vi "ExposeFromObjectMap.vi"(8 "Allow Variant Values (f)":bool, 10 "Object Map":T1[](array[typedef]), 11 "Type (or value to update)":variant) -> (3 "Value":variant)   [LabVIEW 2017]
uses:
  ExposeObjectMapNamepathData.ctl
  ExposeObjectMapDataTypeEnum.ctl
  ExposeObjectMapContainerTypeEnum.ctl
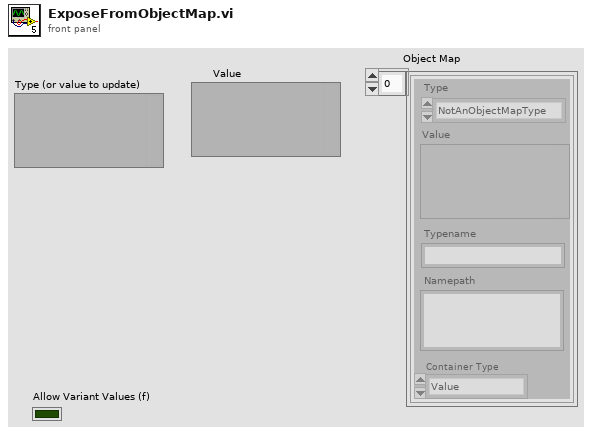
[diagram p1: front panel]
types:
  T1 = typedef "ExposeObjectMapNamepathData.ctl" = cluster{"Type":T2, "Value":variant, "Namepath":string, "Typename":string, "Container Type":T3}
  T2 = typedef "ExposeObjectMapDataTypeEnum.ctl" = enum16{"NotAnObjectMapType", "Real", "Complex", "String", "Boolean"}
  T3 = typedef "ExposeObjectMapContainerTypeEnum.ctl" = enum16{"Value", "Array", "Waveform"}
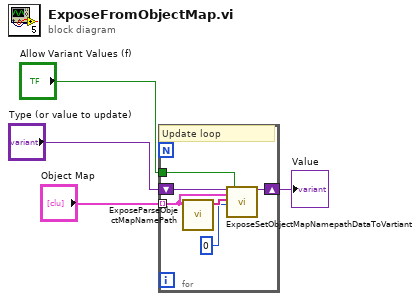
[diagram p0: block diagram]
diagram:
  n1 = for {
    tunnel: "Object Map" -> [w6] mode=indexing
    shift-right: [w8] -> w3
    shift-left: "Type (or value to update)" -> [w9]
    tunnel: "Allow Variant Values (f)" -> [w5]
    # "Update loop"
    n2 = call "ExposeParseObjectMapNamePath.vi"("MatlabDataBundle"=w6) -> ("Name parts array"=w10:string[])  [unwired: 10 in]
    n3 = call "ExposeSetObjectMapNamepathDataToVartiant.vi"("Type (or value to update)"=w9, "MatlabDataBundle"=w6, "NamePath"=w10, "Namepath Index"=0 ("curNameIndex"), "Allow Variant Values (f)"=w5) -> ("Value"=w8:variant)  [unwired: 14 in]
  }
  "Value" <- w3
